vi "Not A DSF Configuration Data Refnum.vi"(1 "dsf refnum":T1) -> (0 "not a dsf refnum":bool)   [LabVIEW 2017, in "DSF Configuration API.lvlib"]
doc: "Determines whether a configuration data dsf refnum is valid."
uses:
  DSF Configuration API.lvlib
  Controls/DSF Config Data RefNum.ctl
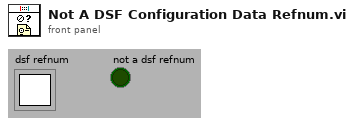
[diagram p1: front panel]
types:
  T1 = typedef "DSF Configuration API.lvlib/DSF Config Data RefNum.ctl" = refnum<k1>
  T2 = typedef "DSF Configuration API.lvlib/DSF Configuration Reference.ctl" = refnum<data-value>
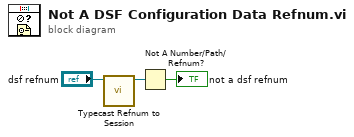
[diagram p0: block diagram]
diagram:
  n1 = call "Typecast Refnum to Session.vi"("dsf refnum in"="dsf refnum") -> ("DSF Configuration Session out"=w2:T2)  [unwired: 10 in]
  n2 = Not A Number/Path/Refnum?(number/path/refnum=w2) -> (NaN/Path/Refnum?=→"not a dsf refnum":bool)
